vi "Read ID.vi"(8 "error in (no error)":errorcluster, 11 "Calibrator in":refnum<class "Calibrator.lvclass">) -> (0 "error out":errorcluster, 3 "Calibrator out":refnum<class "Calibrator.lvclass">)   [LabVIEW 2015, in "Calibrator.lvclass"]
doc: "VI used to Read Hardware ID"
uses:
  Calibrator.lvclass
  <instrlib>/Fluke 5XXX Series Multicalibrators/Fluke 5XXX Series Multicalibrators.lvlib
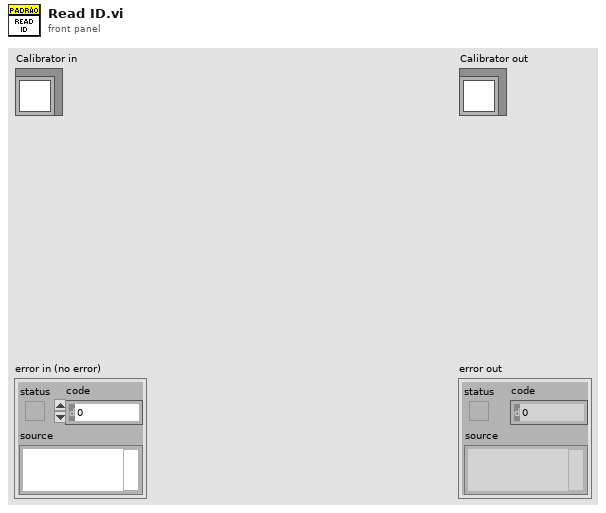
[diagram p1: front panel]
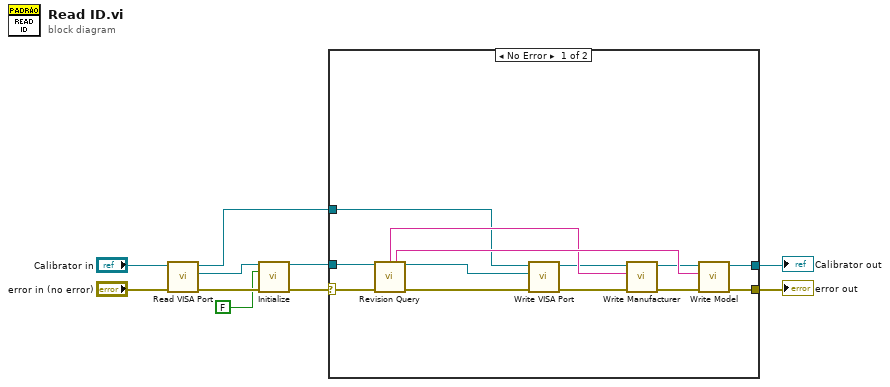
[diagram p0: block diagram]
diagram:
  n1 = call-dynamic "Read VISA Port.vi"("error in (no error)"="error in (no error)", "Device in"="Calibrator in") -> ("error out"=w3:errorcluster, "VISA Port"=w2:refnum<visa-resource-name>, "Device out"=w10:refnum<class "Calibrator.lvclass">)  [unwired: 7 in]
  n2 = call <instrlib>:"Initialize.vi"("VISA resource name"=w2, "ID Query (T: Check)"=FALSE, "error in (no error)"=w3) -> ("VISA resource name out"=w4:refnum<visa-resource-name>, "error out"=w5:errorcluster)  [unwired: 11 in]
  n3 = case shown="No Error" w5 {
    selector: w5 -> [w22 w24]
    tunnel: w4 -> [w23 _]
    tunnel: w10 -> [w15 w25]
    tunnel: [w17 w24] -> w6
    tunnel: [w18 w25] -> w7
    frame No Error {
      n4 = call <instrlib>:"Revision Query.vi"("VISA resource name"=w23, "error in (no error)"=w22) -> ("Fabricante"=w16:string, "Modelo"=w21:string, "VISA resource name out"=w14:refnum<visa-resource-name>, "error out"=w12:errorcluster)  [unwired: 10 in]
      n5 = call-dynamic "Write VISA Port.vi"("error in (no error)"=w12, "VISA Port"=w14, "Device in"=w15) -> ("error out"=w11:errorcluster, "Device out"=w13:refnum<class "Calibrator.lvclass">)  [unwired: 7 in]
      n6 = call-dynamic "Write Manufacturer.vi"("error in (no error)"=w11, "Manufacturer"=w16, "Device in"=w13) -> ("error out"=w20:errorcluster, "Device out"=w19:refnum<class "Calibrator.lvclass">)  [unwired: 7 in]
      n7 = call-dynamic "Write Model.vi"("error in (no error)"=w20, "Model"=w21, "Device in"=w19) -> ("error out"=w17:errorcluster, "Device out"=w18:refnum<class "Calibrator.lvclass">)  [unwired: 7 in]
    }
    frame Error {
    }
  }
  "error out" <- w6
  "Calibrator out" <- w7
